vi "TDMS_Write.vi"(8 "2D data array":string[][](array[string])) -> ()   [LabVIEW 2015]
uses:
  Robot Global Data.vi
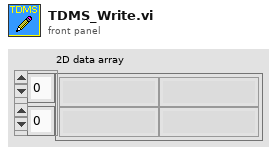
[diagram p1: front panel]
types:
  T1 = enum16{"open", "open or create", "create or replace", "create", "open (read-only)"}
  T2 = cluster{"Record?":bool, "Current File":string, "Run script?":bool, "Stop recording?":bool, "Stop script?":bool}
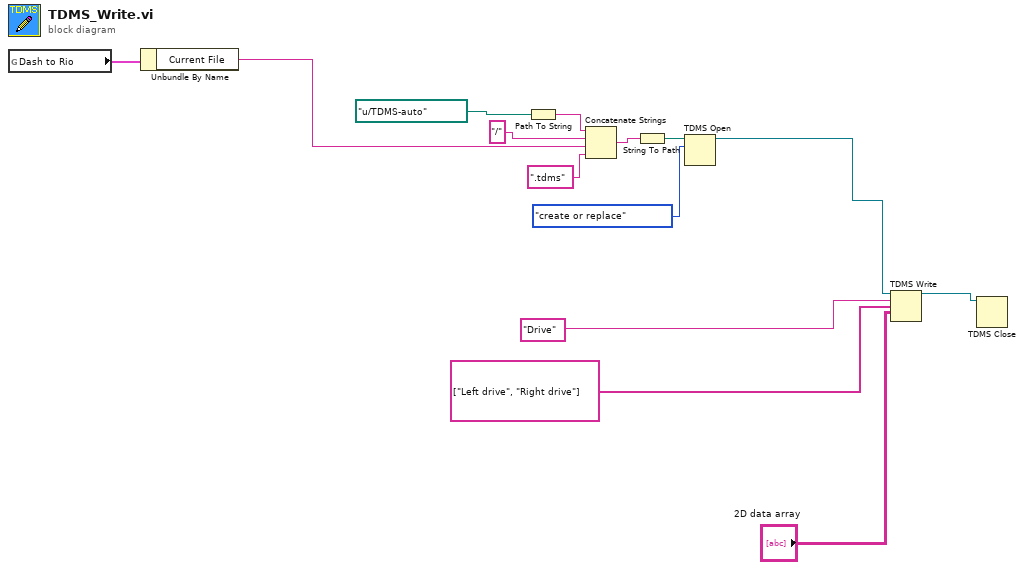
[diagram p0: block diagram]
diagram:
  n1 = global read "Robot Global Data.vi" "Dash to Rio"() -> (w4:T2)
  n2 = Unbundle By Name(w4) -> ("Current File"=w2:string)
  n3 = Path To String(path=path "u:/TDMS-auto" ("file path 3")) -> (string=w12:string)
  n4 = Concatenate Strings(w12, "/" ("TDMS file name"), w2, ".tdms" ("string")) -> (w6:string)
  n5 = String To Path(string=w6) -> (path=w9:path)
  n6 = TDMS Open(10:T1."create or replace" ("operation (0:open)"), 11:w9) -> (3:w8:refnum<k34>)  [unwired: 5 in, 1 out]
  n7 = TDMS Write(0:w8, 5:"Drive" ("group name in"), 7:string[] ["Left drive", "Right drive"] ("channel name(s) in"), 9:"2D data array") -> (4:w7:refnum<k34>)  [unwired: 2 in, 3 out]
  n8 = TDMS Close(11:w7) -> ()  [unwired: 1 in, 2 out]
